vi "Nespresso.vi"() -> ()   [LabVIEW 2022 SP3]
panel:
  out "Cafés corespondants à l'intensité choisie":string[][](array[string])
  in  "Numeric":dbl
  in  "val":bool
  in  "Reset":bool
  in  "Stop program":bool
  in  "New selection ?":bool
  in  "Volume de la tasse":string(combo)
  in  "Coffee extraction 2":bool
  out "Intensité des cafés correspondants à vos critères":bool[][](array[boolean])
  out "Cafés correspondants à vos critères":string[](array[string])
  in  "Intensité désirée":bool[](array[boolean])=[FALSE, FALSE, FALSE, FALSE, FALSE, FALSE, FALSE, FALSE, FALSE, FALSE, FALSE, FALSE]
  in  "Coffee extraction":bool
  in  "Extraction par intensité":bool
  in  "Extraction par volume de la tasse":bool
  out "Numeric 2":i32
  in  "Nom":string
  in  "Prénom":string
  in  "Mot de passe":string
  out "Identification correcte":bool
  out "identification message":string
  out "String":string
  in  "Boolean":bool
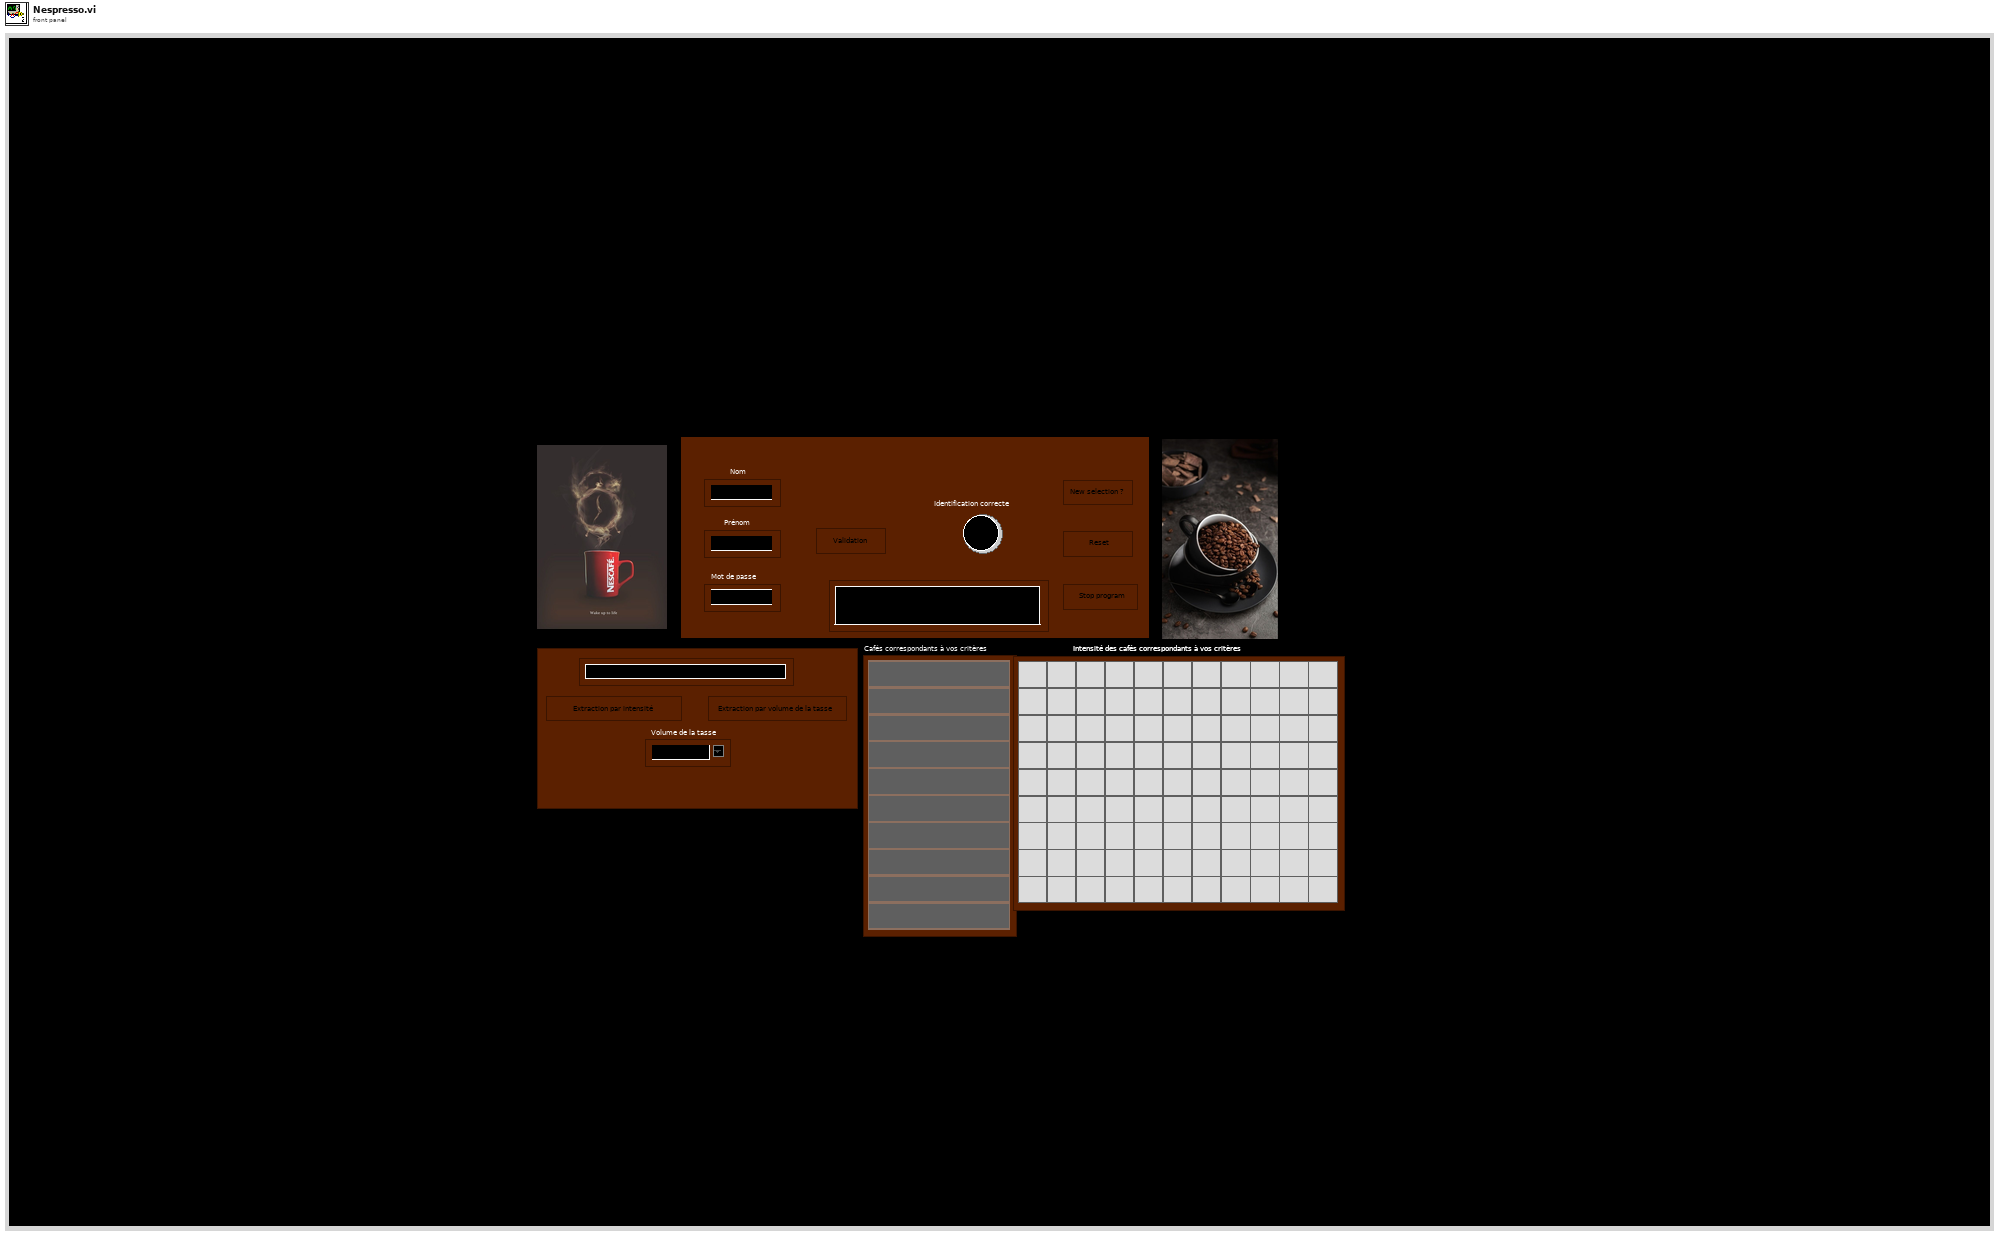
[diagram p1: front panel]
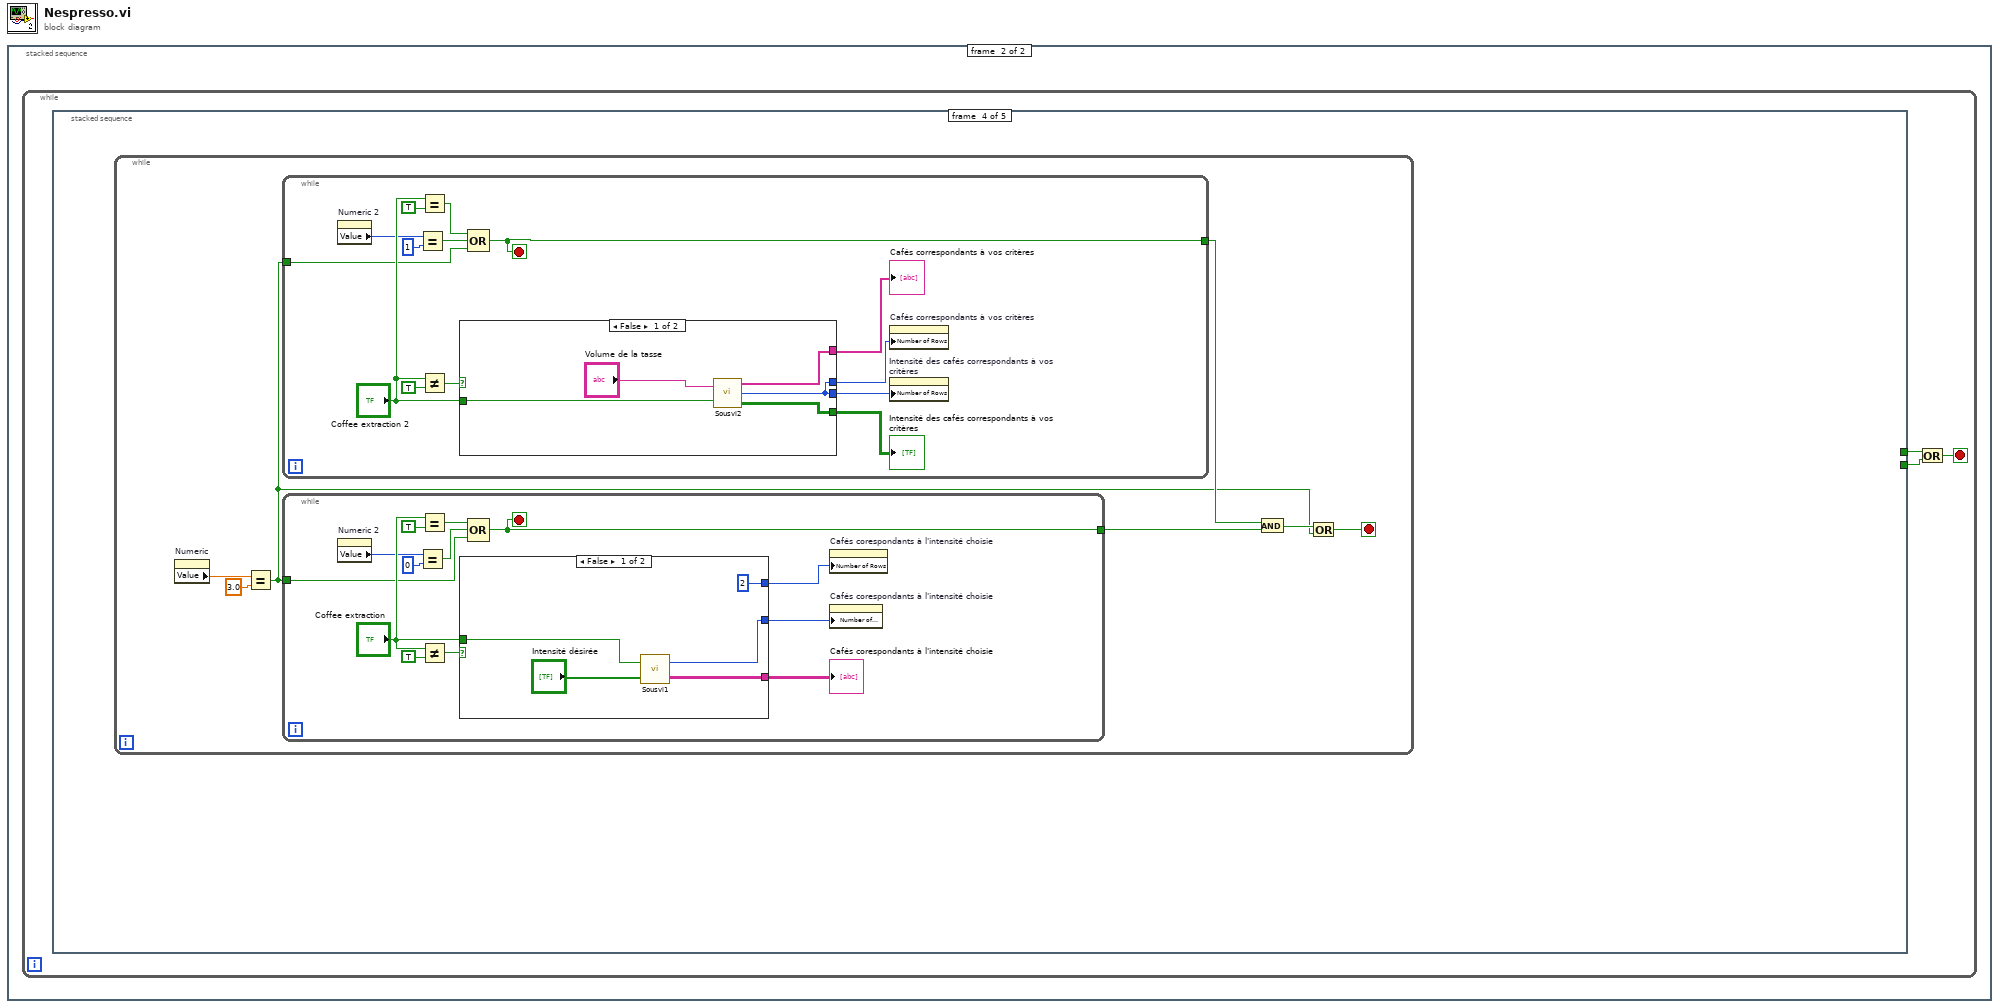
[diagram p0: block diagram]
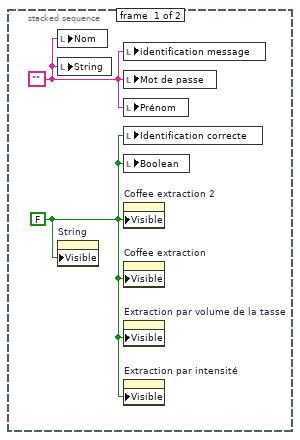
[diagram p2: hidden frame]
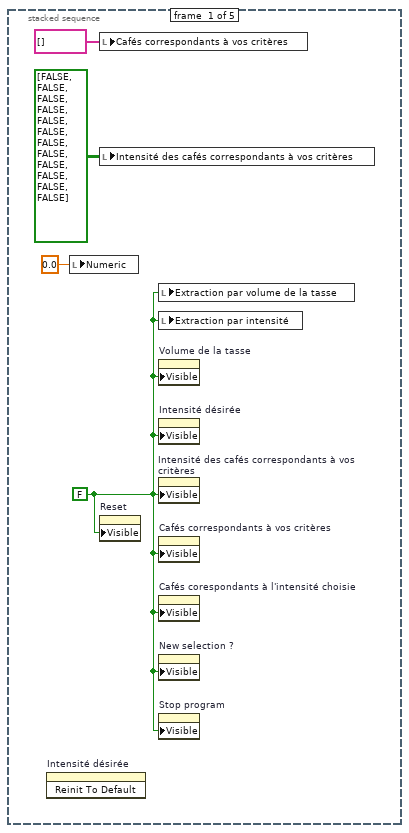
[diagram p3: hidden frame]
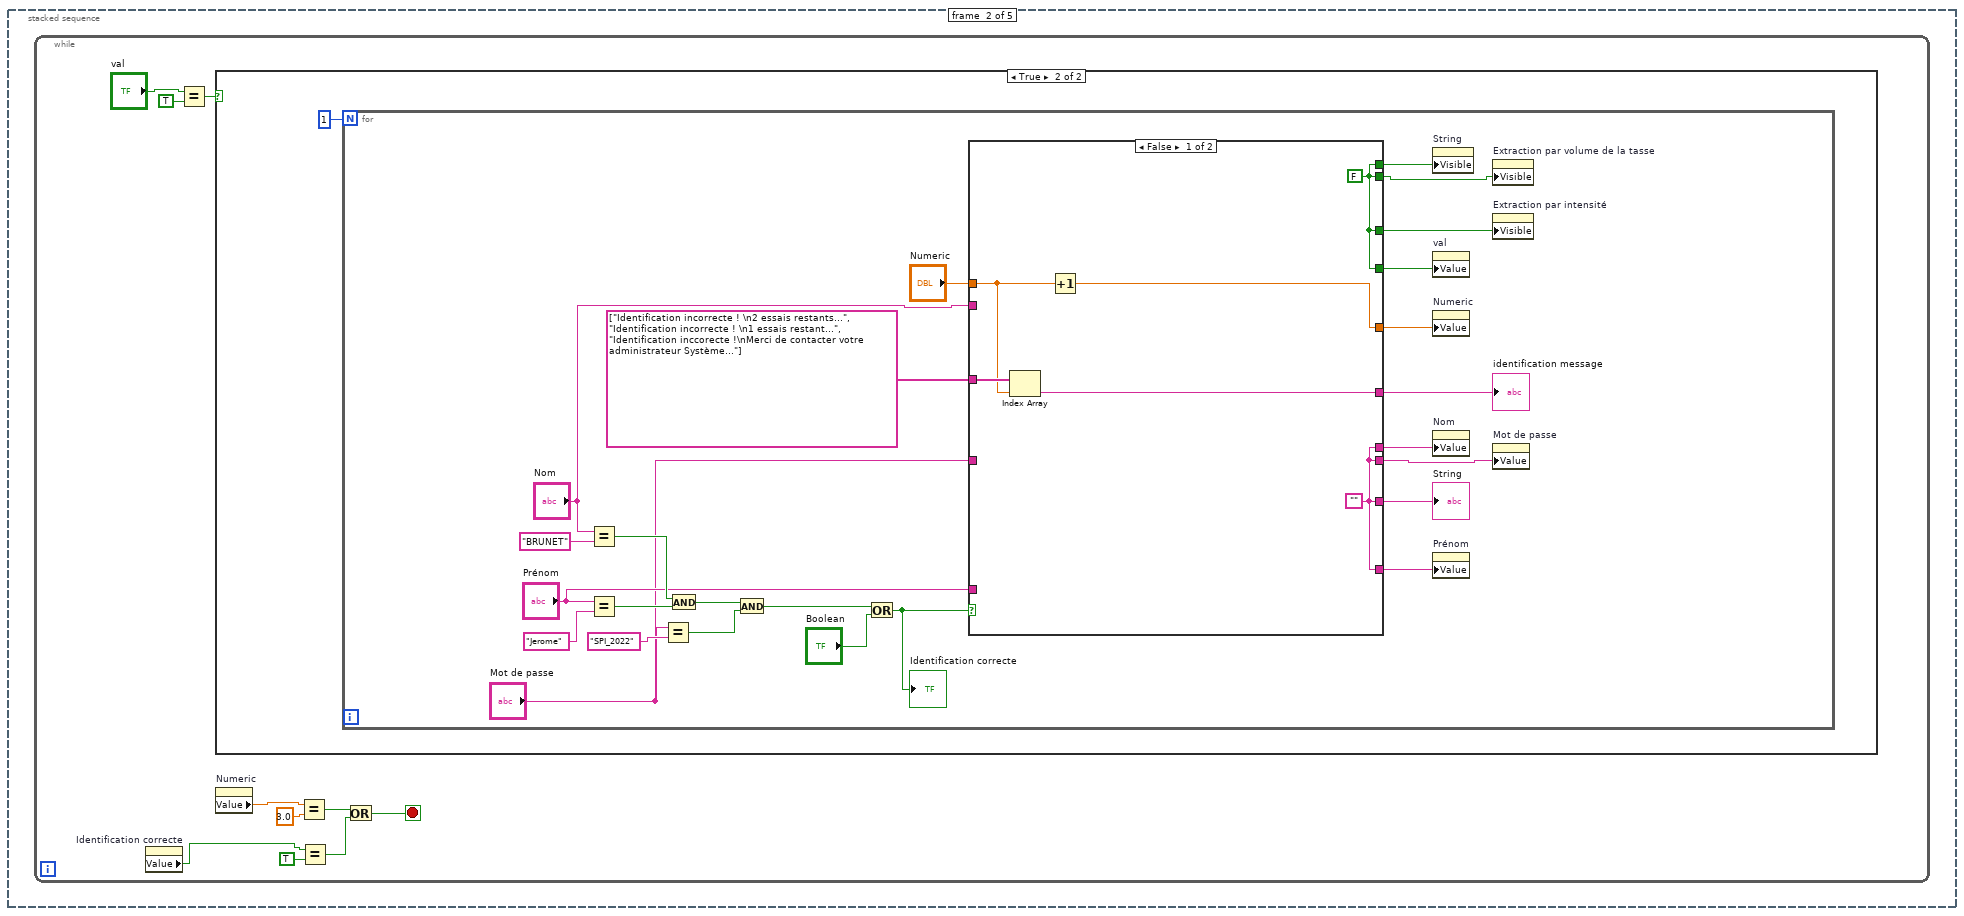
[diagram p4: hidden frame]
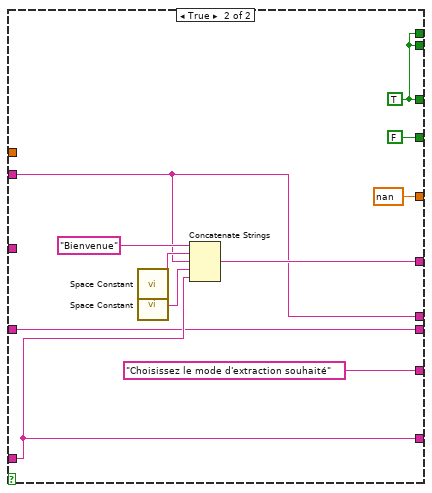
[diagram p6: hidden frame]
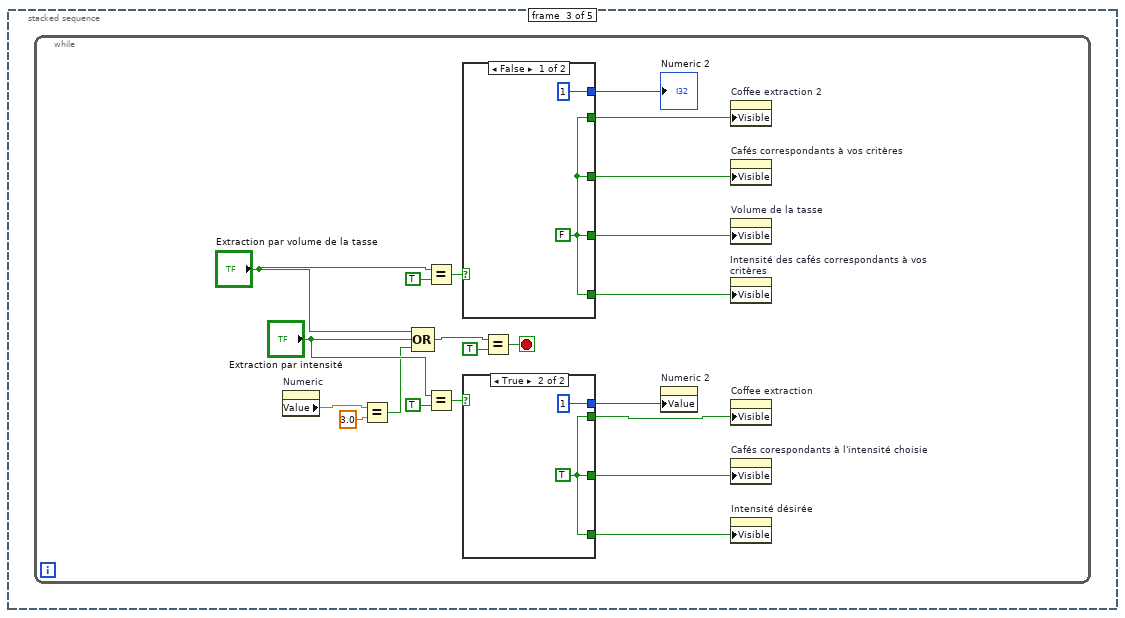
[diagram p7: hidden frame]
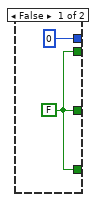
[diagram p8: hidden frame]
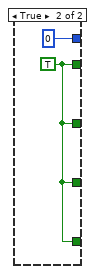
[diagram p9: hidden frame]
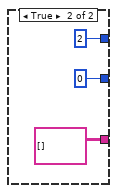
[diagram p10: hidden frame]
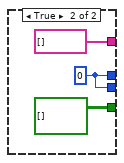
[diagram p11: hidden frame]
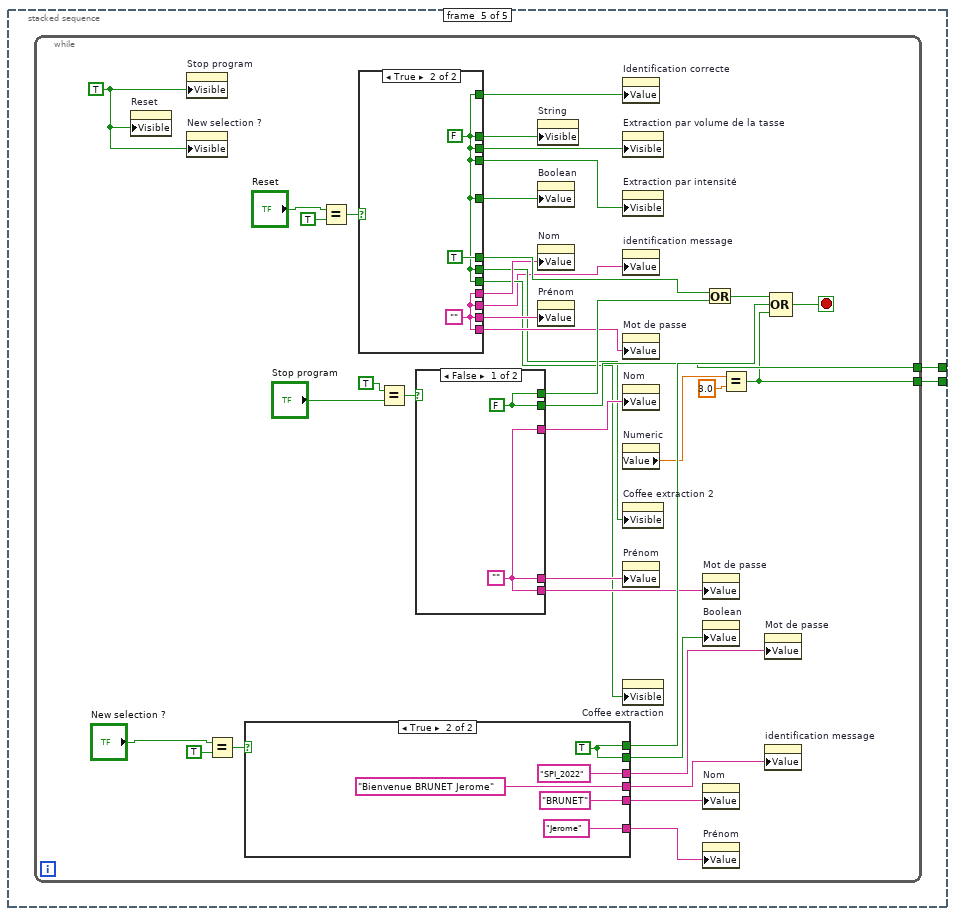
[diagram p12: hidden frame]
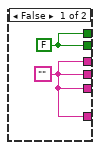
[diagram p13: hidden frame]
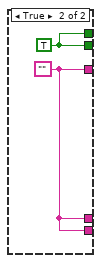
[diagram p14: hidden frame]
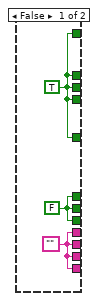
[diagram p15: hidden frame]
diagram:
  n1 = stacked-sequence {
    frame #0 {
      w1 = FALSE
      w2 = ""
      n2 = local write "Nom"(w2) -> ()
      n3 = local write "String"(w2) -> ()
      n4 = property on="String" class="Str"("Visible"=w1) -> ()  [unwired: 2 in, 2 out]
      n5 = local write "identification message"(w2) -> ()
      n6 = local write "Mot de passe"(w2) -> ()
      n7 = local write "Prénom"(w2) -> ()
      n8 = local write "Identification correcte"(w1) -> ()
      n9 = local write "Boolean"(w1) -> ()
      n10 = property on="Coffee extraction 2" class="Bool"("Visible"=w1) -> ()  [unwired: 2 in, 2 out]
      n11 = property on="Coffee extraction" class="Bool"("Visible"=w1) -> ()  [unwired: 2 in, 2 out]
      n12 = property on="Extraction par volume de la tasse" class="Bool (strict)"("Visible"=w1) -> ()  [unwired: 2 in, 2 out]
      n13 = property on="Extraction par intensité" class="Bool (strict)"("Visible"=w1) -> ()  [unwired: 2 in, 2 out]
    }
    frame #1 {
      n14 = while {
        stop <- w5 stop-if-true
        n15 = stacked-sequence {
          tunnel: [_ _ _ _ w142] -> w4
          tunnel: [_ _ _ _ w143] -> w3
          frame #0 {
            w6 = FALSE
            n16 = invoke on="Intensité désirée" class="Arr" method="Reinit To Default"() -> ()  [unwired: 3 in, 3 out]
            n17 = local write "Numeric"(0.0 ("Numeric")) -> ()
            n18 = local write "Cafés correspondants à vos critères"(string[] [] ("subarray")) -> ()
            n19 = local write "Intensité des cafés correspondants à vos critères"(bool[][] [[FALSE], [FALSE], [FALSE], [FALSE], [FALSE], [FALSE], [FALSE], [FALSE], [FALSE], [FALSE], [FALSE], [FALSE]] ("Array 2")) -> ()
            n20 = property on="Reset" class="Bool"("Visible"=w6) -> ()  [unwired: 2 in, 2 out]
            n21 = local write "Extraction par volume de la tasse"(w6) -> ()
            n22 = local write "Extraction par intensité"(w6) -> ()
            n23 = property on="Volume de la tasse" class="CmbBox"("Visible"=w6) -> ()  [unwired: 2 in, 2 out]
            n24 = property on="Intensité désirée" class="Arr"("Visible"=w6) -> ()  [unwired: 2 in, 2 out]
            n25 = property on="Intensité des cafés correspondants à vos critères" class="Arr (strict)"("Visible"=w6) -> ()  [unwired: 2 in, 2 out]
            n26 = property on="Cafés correspondants à vos critères" class="Arr (strict)"("Visible"=w6) -> ()  [unwired: 2 in, 2 out]
            n27 = property on="Cafés corespondants à l'intensité choisie" class="Arr (strict)"("Visible"=w6) -> ()  [unwired: 2 in, 2 out]
            n28 = property on="New selection ?" class="Bool"("Visible"=w6) -> ()  [unwired: 2 in, 2 out]
            n29 = property on="Stop program" class="Bool"("Visible"=w6) -> ()  [unwired: 2 in, 2 out]
          }
          frame #1 {
            n30 = while {
              stop <- w10 stop-if-true
              n31 = property on="Identification correcte" class="Bool (strict)"() -> ("Value"=w17:bool)  [unwired: 2 in, 2 out]
              n32 = Equal?(x="val", y=TRUE) -> (x = y?=w15:bool)
              n33 = case shown="True" w15 {
                frame False {
                }
                frame True {
                  n34 = for {
                    N: 1 -> [_]
                    n35 = Equal?(x="Nom", y="BRUNET") -> (x = y?=w42:bool)
                    n36 = Equal?(x="Prénom", y="Jerome") -> (x = y?=w41:bool)
                    n37 = Equal?(x="Mot de passe", y="SPI_2022") -> (x = y?=w33:bool)
                    n38 = And(x=w42, y=w41) -> (x .and. y?=w34:bool)
                    n39 = And(x=w34, y=w33) -> (x .and. y?=w25:bool)
                    n40 = Or(x=w25, y="Boolean") -> (x .or. y?=w31:bool)
                    "Identification correcte" <- w31
                    n41 = case shown="False" w31 {
                      tunnel: "Nom" -> [_ w56]
                      tunnel: [w48 w60] -> w40
                      tunnel: [w51 "Choisissez le mode d'extraction souhaité"] -> w37
                      tunnel: "Prénom" -> [_ w57]
                      tunnel: [w46 w52] -> w36
                      tunnel: [w46 w52] -> w35
                      tunnel: [w51 w56] -> w30
                      tunnel: [w51 w57] -> w29
                      tunnel: [w51 w55] -> w28
                      tunnel: "Mot de passe" -> [_ w55]
                      tunnel: [w46 FALSE] -> w26
                      tunnel: "Numeric" -> [w47 _]
                      tunnel: [w49 nan] -> w23
                      tunnel: string[] ["Identification incorrecte ! \n2 essais restants...", "Identification incorrecte ! \n1 essais restant...", "Identification inccorecte !\nMerci de contacter votre administrateur Système..."] -> [w50 _]
                      tunnel: [w46 w52] -> w21
                      frame False {
                        w46 = FALSE
                        w51 = ""
                        n42 = Index Array(array=w50, index=w47) -> (element=w48:string)
                        n43 = Increment(x=w47) -> (x+1=w49:dbl)
                      }
                      frame True {
                        w52 = TRUE
                        n44 = call <vilib>:"Space Constant.vi"() -> ("String"=w61:string)
                        n45 = call <vilib>:"Space Constant.vi"() -> ("String"=w58:string)
                        n46 = Concatenate Strings("Bienvenue", w61, w56, w58, w57) -> (w60:string)
                      }
                    }
                    "identification message" <- w40
                    "String" <- w37
                    n47 = property on="String" class="Str"("Visible"=w21) -> ()  [unwired: 2 in, 2 out]
                    n48 = property on="val" class="Bool (strict)"("Value"=w26) -> ()  [unwired: 2 in, 2 out]
                    n49 = property on="Numeric" class="DigNum (strict)"("Value"=w23) -> ()  [unwired: 2 in, 2 out]
                    n50 = property on="Nom" class="Str"("Value"=w30) -> ()  [unwired: 2 in, 2 out]
                    n51 = property on="Prénom" class="Str"("Value"=w29) -> ()  [unwired: 2 in, 2 out]
                    n52 = property on="Extraction par volume de la tasse" class="Bool (strict)"("Visible"=w35) -> ()  [unwired: 2 in, 2 out]
                    n53 = property on="Extraction par intensité" class="Bool (strict)"("Visible"=w36) -> ()  [unwired: 2 in, 2 out]
                    n54 = property on="Mot de passe" class="Str"("Value"=w28) -> ()  [unwired: 2 in, 2 out]
                  }
                }
              }
              n55 = property on="Numeric" class="DigNum (strict)"() -> ("Value"=w14:dbl)  [unwired: 2 in, 2 out]
              n56 = Equal?(x=w14, y=3.0) -> (x = y?=w11:bool)
              n57 = Equal?(x=w17, y=TRUE) -> (x = y?=w12:bool)
              n58 = Or(x=w11, y=w12) -> (x .or. y?=w10:bool)
            }
          }
          frame #2 {
            n59 = while {
              stop <- w75 stop-if-true
              n60 = property on="Numeric" class="DigNum (strict)"() -> ("Value"=w66:dbl)  [unwired: 2 in, 2 out]
              n61 = Equal?(x=w66, y=3.0) -> (x = y?=w64:bool)
              n62 = Compound Arithmetic op=OR("Extraction par volume de la tasse", "Extraction par intensité", w64) -> (w77:bool)
              n63 = Equal?(x="Extraction par volume de la tasse", y=TRUE) -> (x = y?=w83:bool)
              n64 = Equal?(x="Extraction par intensité", y=TRUE) -> (x = y?=w80:bool)
              n65 = case shown="False" w83 {
                tunnel: [w89 w91] -> w72
                tunnel: [w89 w91] -> w73
                tunnel: [w89 w91] -> w71
                tunnel: [w89 w91] -> w69
                tunnel: [1 0] -> w68
                frame False {
                  w89 = FALSE
                }
                frame True {
                  w91 = TRUE
                }
              }
              "Numeric 2" <- w68
              n66 = case shown="True" w80 {
                tunnel: [w85 w87] -> w74
                tunnel: [w85 w87] -> w63
                tunnel: [w85 w87] -> w70
                tunnel: [0 1] -> w67
                frame False {
                  w85 = FALSE
                }
                frame True {
                  w87 = TRUE
                }
              }
              n67 = Equal?(x=w77, y=TRUE) -> (x = y?=w75:bool)
              n68 = property on="Numeric 2" class="DigNum (strict)"("Value"=w67) -> ()  [unwired: 2 in, 2 out]
              n69 = property on="Coffee extraction 2" class="Bool"("Visible"=w69) -> ()  [unwired: 2 in, 2 out]
              n70 = property on="Cafés correspondants à vos critères" class="Arr (strict)"("Visible"=w71) -> ()  [unwired: 2 in, 2 out]
              n71 = property on="Volume de la tasse" class="CmbBox"("Visible"=w73) -> ()  [unwired: 2 in, 2 out]
              n72 = property on="Intensité des cafés correspondants à vos critères" class="Arr (strict)"("Visible"=w72) -> ()  [unwired: 2 in, 2 out]
              n73 = property on="Coffee extraction" class="Bool"("Visible"=w70) -> ()  [unwired: 2 in, 2 out]
              n74 = property on="Cafés corespondants à l'intensité choisie" class="Arr (strict)"("Visible"=w63) -> ()  [unwired: 2 in, 2 out]
              n75 = property on="Intensité désirée" class="Arr"("Visible"=w74) -> ()  [unwired: 2 in, 2 out]
            }
          }
          frame #3 {
            n76 = while {
              stop <- w93 stop-if-true
              n77 = property on="Numeric" class="DigNum (strict)"() -> ("Value"=w96:dbl)  [unwired: 2 in, 2 out]
              n78 = Equal?(x=w96, y=3.0) -> (x = y?=w92:bool)
              n79 = while {
                tunnel: [w124] -> w98
                tunnel: w92 -> [w122]
                stop <- w124 stop-if-true
                n80 = property on="Numeric 2" class="DigNum (strict)"() -> ("Value"=w123:i32)  [unwired: 2 in, 2 out]
                n81 = Equal?(x=w123, y=1) -> (x = y?=w125:bool)
                n82 = Equal?(x="Coffee extraction 2", y=TRUE) -> (x = y?=w127:bool)
                n83 = Not Equal?(x="Coffee extraction 2", y=TRUE) -> (x != y?=w131:bool)
                n84 = case shown="False" w131 {
                  tunnel: "Coffee extraction 2" -> [w137 _]
                  tunnel: [w135 bool[][] [] ("Array")] -> w128
                  tunnel: [w136 string[] [] ("subarray")] -> w129
                  tunnel: [w134 w139] -> w121
                  tunnel: [w134 w139] -> w120
                  frame False {
                    n85 = call "Sousvi2.vi"("Combo Box 2"="Volume de la tasse", "Coffee extraction"=w137) -> ("subarray"=w136:string[], "Numeric"=w134:i32, "Array"=w135:bool[][])
                  }
                  frame True {
                    w139 = 0
                  }
                }
                "Intensité des cafés correspondants à vos critères" <- w128
                "Cafés correspondants à vos critères" <- w129
                n86 = Compound Arithmetic op=OR(w127, w125, w122) -> (w124:bool)
                n87 = property on="Cafés correspondants à vos critères" class="Arr (strict)"("Number of Rows"=w121) -> ()  [unwired: 2 in, 2 out]
                n88 = property on="Intensité des cafés correspondants à vos critères" class="Arr (strict)"("Number of Rows"=w120) -> ()  [unwired: 2 in, 2 out]
              }
              n89 = while {
                tunnel: [w104] -> w97
                tunnel: w92 -> [w102]
                stop <- w104 stop-if-true
                n90 = property on="Numeric 2" class="DigNum (strict)"() -> ("Value"=w103:i32)  [unwired: 2 in, 2 out]
                n91 = Equal?(x=w103, y=0) -> (x = y?=w106:bool)
                n92 = Equal?(x="Coffee extraction", y=TRUE) -> (x = y?=w105:bool)
                n93 = Not Equal?(x="Coffee extraction", y=TRUE) -> (x != y?=w109:bool)
                n94 = case shown="False" w109 {
                  tunnel: "Coffee extraction" -> [w116 _]
                  tunnel: [w114 string[][] [] ("appended array")] -> w101
                  tunnel: [w113 0 ("Nombre de colonnes")] -> w100
                  tunnel: [2 2] -> w99
                  frame False {
                    n95 = call "Sousvi1.vi"("Array"="Intensité désirée", "Coffee extraction"=w116) -> ("appended array"=w114:string[][], "Nombre de colonnes"=w113:i32)
                  }
                  frame True {
                  }
                }
                "Cafés corespondants à l'intensité choisie" <- w101
                n96 = Compound Arithmetic op=OR(w105, w106, w102) -> (w104:bool)
                n97 = property on="Cafés corespondants à l'intensité choisie" class="Arr (strict)"("Number of Rows"=w99) -> ()  [unwired: 2 in, 2 out]
                n98 = property on="Cafés corespondants à l'intensité choisie" class="Arr (strict)"("Number of Columns"=w100) -> ()  [unwired: 2 in, 2 out]
              }
              n99 = And(x=w98, y=w97) -> (x .and. y?=w94:bool)
              n100 = Or(x=w94, y=w92) -> (x .or. y?=w93:bool)
            }
          }
          frame #4 {
            n101 = while {
              tunnel: [w160] -> w143
              tunnel: [w157] -> w142
              stop <- w168 stop-if-true
              w176 = TRUE
              n102 = property on="Reset" class="Bool"("Visible"=w176) -> ()  [unwired: 2 in, 2 out]
              n103 = property on="Stop program" class="Bool"("Visible"=w176) -> ()  [unwired: 2 in, 2 out]
              n104 = property on="New selection ?" class="Bool"("Visible"=w176) -> ()  [unwired: 2 in, 2 out]
              n105 = Equal?(x="New selection ?", y=TRUE) -> (x = y?=w173:bool)
              n106 = case shown="True" w173 {
                tunnel: [w183 w188] -> w166
                tunnel: [w183 w188] -> w164
                tunnel: [w182 "BRUNET"] -> w156
                tunnel: [w182 "Jerome"] -> w155
                tunnel: [w182 "SPI_2022"] -> w154
                tunnel: [w182 "Bienvenue BRUNET Jerome"] -> w144
                frame False {
                  w182 = ""
                  w183 = FALSE
                }
                frame True {
                  w188 = TRUE
                }
              }
              n107 = Equal?(x="Reset", y=TRUE) -> (x = y?=w181:bool)
              n108 = case shown="True" w181 {
                tunnel: [w195 w197] -> w170
                tunnel: [w194 TRUE] -> w167
                tunnel: [w195 w197] -> w165
                tunnel: [w193 w196] -> w163
                tunnel: [w193 w196] -> w162
                tunnel: [w193 w196] -> w161
                tunnel: [w195 w197] -> w150
                tunnel: [w195 w197] -> w149
                tunnel: [w195 w197] -> w148
                tunnel: [w194 w197] -> w147
                tunnel: [w194 w197] -> w146
                tunnel: [w193 w196] -> w145
                frame False {
                  w193 = ""
                  w194 = FALSE
                  w195 = TRUE
                }
                frame True {
                  w196 = ""
                  w197 = FALSE
                }
              }
              n109 = Equal?(x=TRUE, y="Stop program") -> (x = y?=w175:bool)
              n110 = case shown="False" w175 {
                tunnel: [w190 w192] -> w169
                tunnel: [w190 w192] -> w160
                tunnel: [w189 w191] -> w153
                tunnel: [w189 w191] -> w152
                tunnel: [w189 w191] -> w151
                frame False {
                  w189 = ""
                  w190 = FALSE
                }
                frame True {
                  w191 = ""
                  w192 = TRUE
                }
              }
              n111 = property on="String" class="Str"("Visible"=w150) -> ()  [unwired: 2 in, 2 out]
              n112 = property on="Boolean" class="Bool (strict)"("Value"=w165) -> ()  [unwired: 2 in, 2 out]
              n113 = property on="Nom" class="Str"("Value"=w163) -> ()  [unwired: 2 in, 2 out]
              n114 = property on="Prénom" class="Str"("Value"=w162) -> ()  [unwired: 2 in, 2 out]
              n115 = property on="Identification correcte" class="Bool (strict)"("Value"=w170) -> ()  [unwired: 2 in, 2 out]
              n116 = property on="Extraction par volume de la tasse" class="Bool (strict)"("Visible"=w148) -> ()  [unwired: 2 in, 2 out]
              n117 = property on="Extraction par intensité" class="Bool (strict)"("Visible"=w149) -> ()  [unwired: 2 in, 2 out]
              n118 = property on="identification message" class="Str"("Value"=w145) -> ()  [unwired: 2 in, 2 out]
              n119 = property on="Mot de passe" class="Str"("Value"=w161) -> ()  [unwired: 2 in, 2 out]
              n120 = property on="Nom" class="Str"("Value"=w151) -> ()  [unwired: 2 in, 2 out]
              n121 = property on="Numeric" class="DigNum (strict)"() -> ("Value"=w159:dbl)  [unwired: 2 in, 2 out]
              n122 = property on="Coffee extraction 2" class="Bool"("Visible"=w146) -> ()  [unwired: 2 in, 2 out]
              n123 = property on="Prénom" class="Str"("Value"=w153) -> ()  [unwired: 2 in, 2 out]
              n124 = property on="Coffee extraction" class="Bool"("Visible"=w147) -> ()  [unwired: 2 in, 2 out]
              n125 = property on="Mot de passe" class="Str"("Value"=w152) -> ()  [unwired: 2 in, 2 out]
              n126 = property on="Boolean" class="Bool (strict)"("Value"=w164) -> ()  [unwired: 2 in, 2 out]
              n127 = property on="Nom" class="Str"("Value"=w156) -> ()  [unwired: 2 in, 2 out]
              n128 = property on="Prénom" class="Str"("Value"=w155) -> ()  [unwired: 2 in, 2 out]
              n129 = Or(x=w167, y=w169) -> (x .or. y?=w178:bool)
              n130 = Equal?(x=w159, y=3.0) -> (x = y?=w157:bool)
              n131 = property on="Mot de passe" class="Str"("Value"=w154) -> ()  [unwired: 2 in, 2 out]
              n132 = property on="identification message" class="Str"("Value"=w144) -> ()  [unwired: 2 in, 2 out]
              n133 = Compound Arithmetic op=OR(w178, w166, w157) -> (w168:bool)
            }
          }
        }
        n134 = Or(x=w3, y=w4) -> (x .or. y?=w5:bool)
      }
    }
  }
